vi "Launch New Chat Window.vi"(8 "error in (no error)":errorcluster, 11 "Server in":refnum<class "Server.lvclass">) -> (0 "error out":errorcluster, 3 "Server out":refnum<class "Server.lvclass">)   [LabVIEW 2019, in "Server.lvlib" / "Server.lvclass"]
uses:
  Server.lvclass
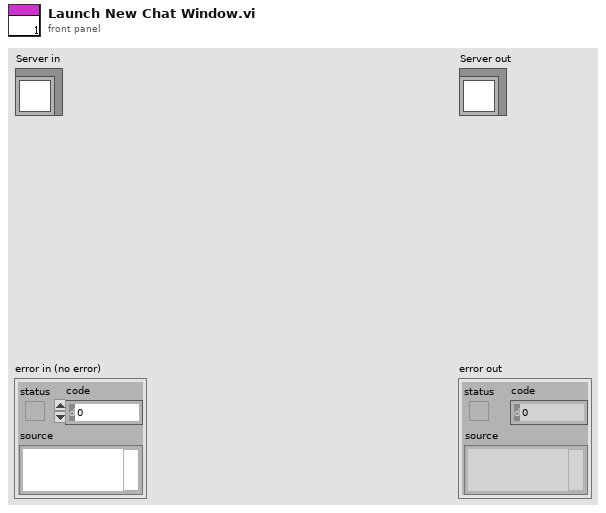
[diagram p1: front panel]
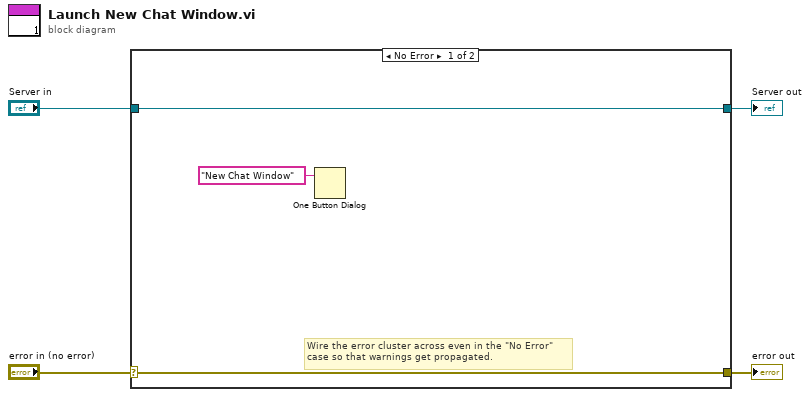
[diagram p0: block diagram]
diagram:
  n1 = case shown="No Error" "error in (no error)" {
    selector: "error in (no error)" -> [w6 w9]
    tunnel: [w6 w9] -> w3
    tunnel: [w7 w8] -> w1
    tunnel: "Server in" -> [w7 w8]
    frame No Error {
      # "Wire the error cluster across even in the \"No Error\"\ncase so that warnings get propagated."
      n2 = One Button Dialog(message="New Chat Window") -> ()  [unwired: 1 in, 1 out]
    }
    frame Error {
    }
  }
  "error out" <- w3
  "Server out" <- w1
